vi "GetScaleCenter.vi"(11 "GraphScale入力":refnum<vi>) -> (3 "数値":dbl)   [LabVIEW 2014]
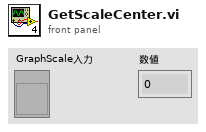
[diagram p1: front panel]
types:
  T1 = typedef "LVRangeTypeDef.ctl" = cluster{"Minimum":dbl, "Maximum":dbl, "Increment":dbl, "Minor Increment":dbl, "Start":dbl}
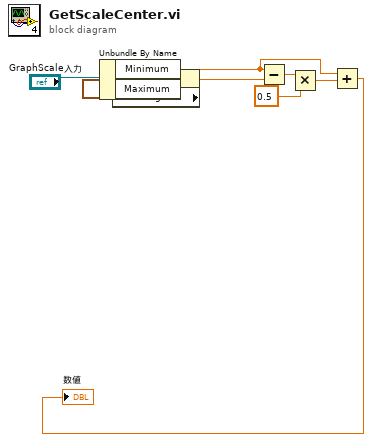
[diagram p0: block diagram]
diagram:
  n1 = property class="GrphScl"(reference="GraphScale入力") -> ("Range"=w8:T1)  [unwired: 1 in, 2 out]
  n2 = Unbundle By Name(w8) -> ("Minimum"=w5:dbl, "Maximum"=w1:dbl)
  n3 = Subtract(x=w5, y=w1) -> (x-y=w2:dbl)
  n4 = Multiply(x=w2, y=0.5) -> (x*y=w4:dbl)
  n5 = Add(x=w5, y=w4) -> (x+y=→"数値":dbl)
